vi "Read code.vi"(8 "error in (no error)":errorcluster, 11 "Parent in":refnum<class "Parent.lvclass">) -> (0 "error out":errorcluster, 2 "code":dbl, 3 "Parent out":refnum<class "Parent.lvclass">)   [LabVIEW 2024, in "Parent.lvclass"]
uses:
  Parent.lvclass
  Parent.lvclass/Parent.ctl
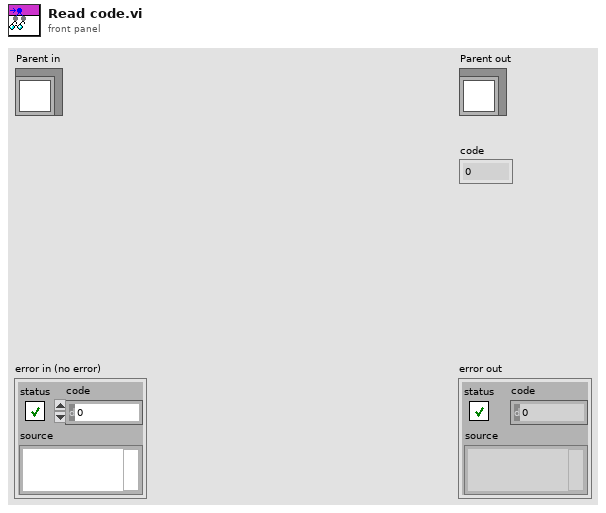
[diagram p1: front panel]
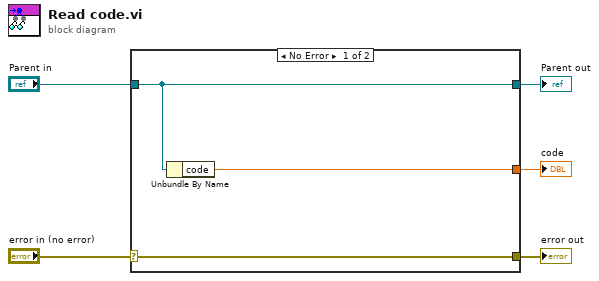
[diagram p0: block diagram]
diagram:
  n1 = case shown="No Error" "error in (no error)" {
    selector: "error in (no error)" -> [w8 w9]
    tunnel: [w8 w9] -> w4
    tunnel: [w7 w10] -> w2
    tunnel: "Parent in" -> [w7 w10]
    tunnel: [w6 _] -> w1
    frame No Error {
      n2 = Unbundle By Name(w7) -> ("code"=w6:dbl)
    }
    frame Error {
    }
  }
  "error out" <- w4
  "Parent out" <- w2
  "code" <- w1
